vi "cam_entropy_trigger.vi"() -> ()   [LabVIEW 2015]
uses:
  <vilib>/userdefined/High Color/IMAQdx.ctl
  <vilib>/vision/driver/IMAQdx.llb/IMAQdx Acquisition Mode.ctl
  <vilib>/vision/driver/NI_Vision_Acquisition_Software.lvlib
  <vilib>/Analysis/NI_AALBase.lvlib
panel:
  in  "Image Name":string
  in  "File Path":path
  out "buffer #":u32
  out "loop count":i32
  in  "Manual Trigger":bool
  in  "error in":errorcluster
  in  "IMAQdx Session":T1="cam0"
  out "Camera Image":T2(plugin-control)
  in  "stop":bool
  out "Skip Frame":bool
  out "Trigger":bool
  out "Abs Entropy":dbl(graph)
  in  "Entropy Threshold":dbl=0.1
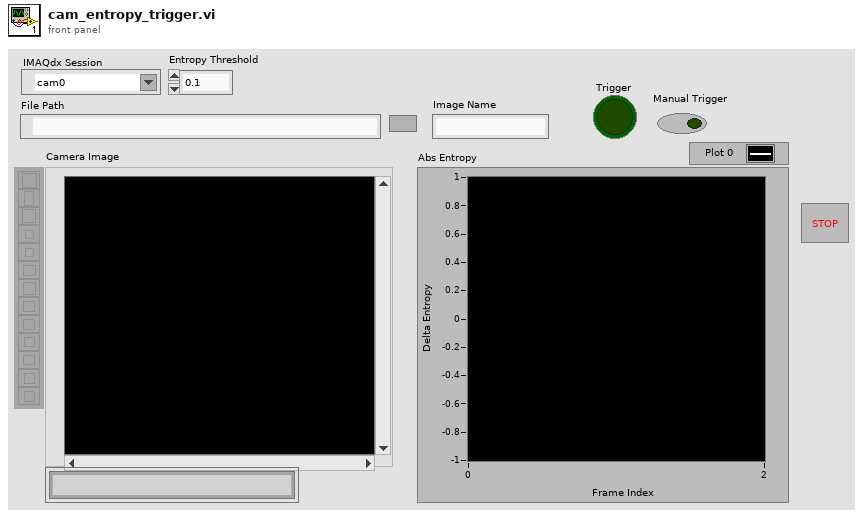
[diagram p1: front panel]
types:
  T1 = typedef "IMAQdx.ctl" = refnum<k21>
  T2 = typedef "IMAQ Image.ctl" = refnum<image>
  T3 = typedef "NI_Vision_Acquisition_Software.lvlib/IMAQdx Acquisition Mode.ctl" = enum32{"One Shot", "Continuous"}
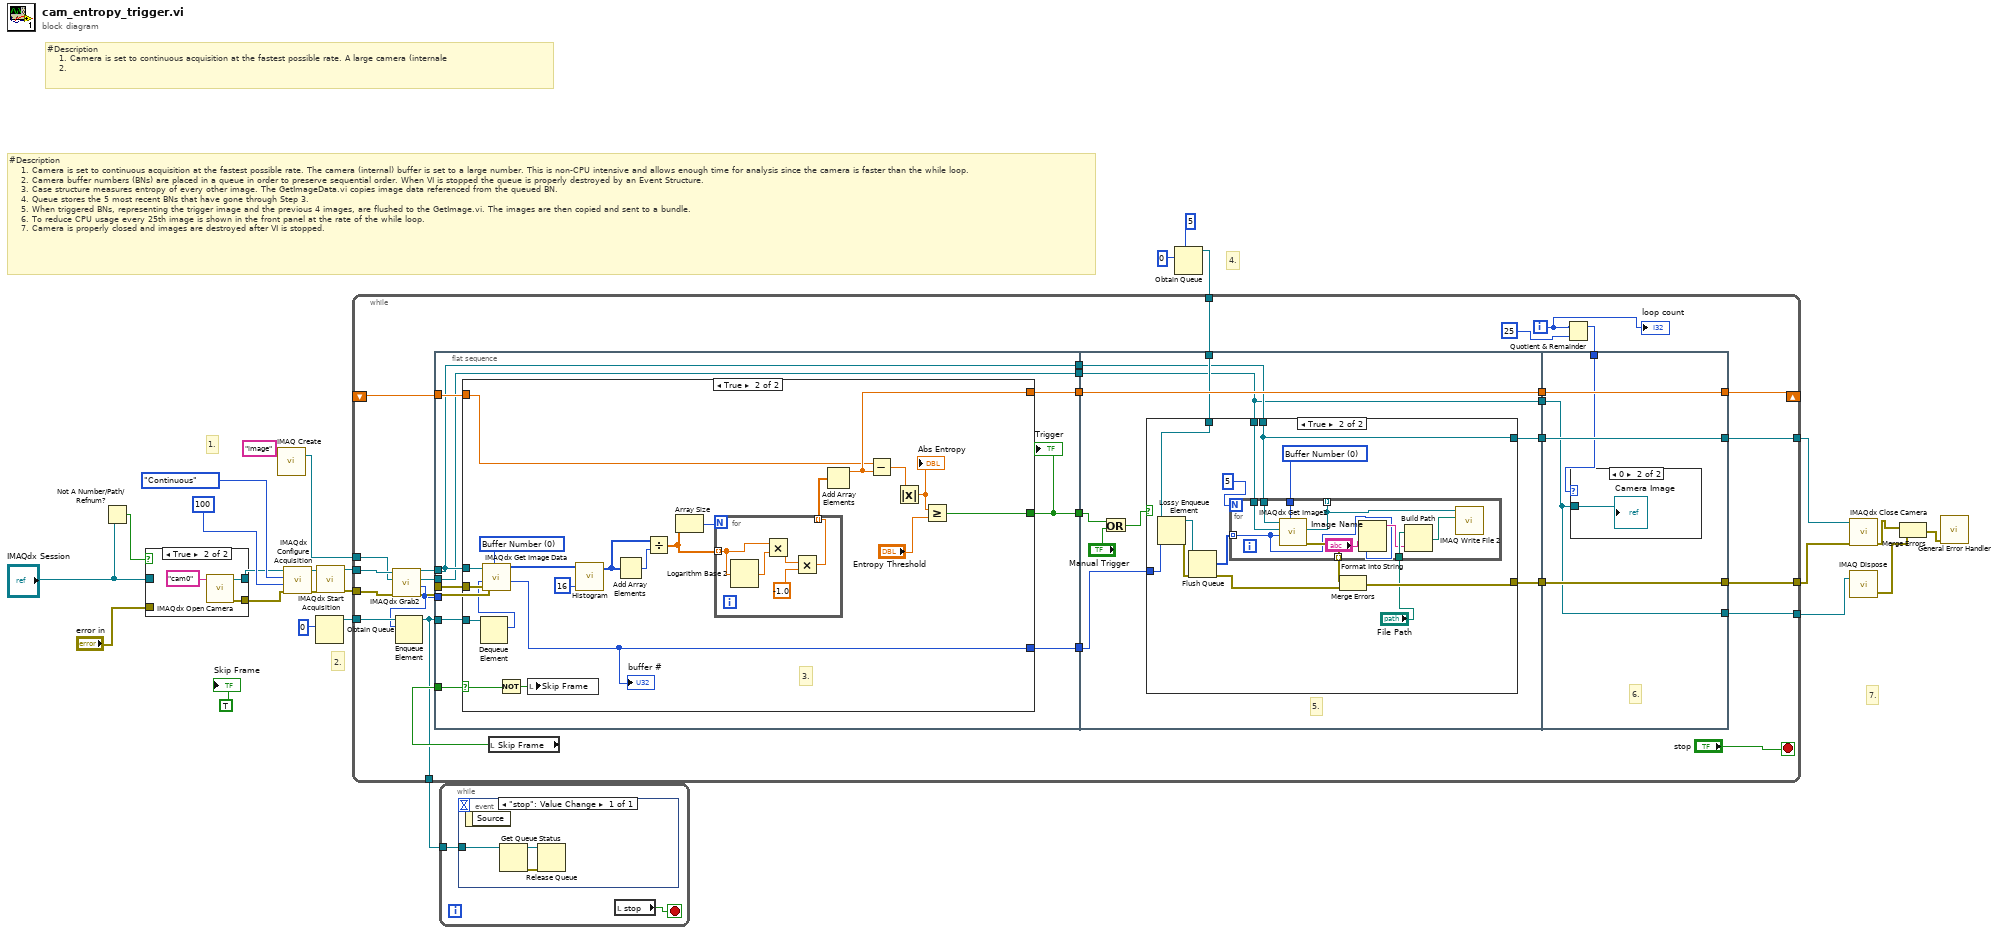
[diagram p0: block diagram]
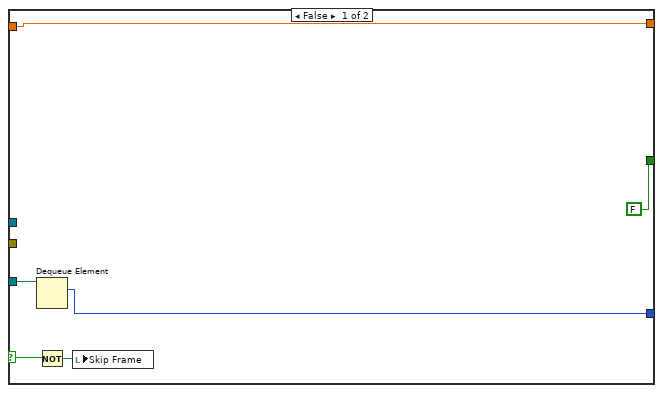
[diagram p3: hidden frame]
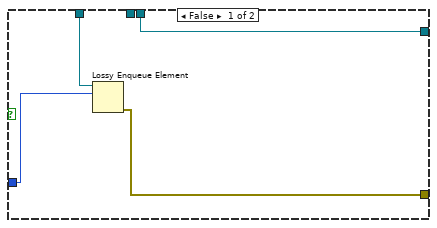
[diagram p4: hidden frame]
diagram:
  # "#Description\n    1. Camera is set to continuous acquisition at the fastest possible rate. The camera (internal) buffer is set to a large number. This is non-CPU intensive and allows enough time for analysis since the camera is faster than the while loop.\n    2. Camera buffer numbers (BNs) are placed in a queue in order to preserve sequential order. When VI is stopped the queue is properly destroyed by an Event Structure.\n    3. Case structure measures entropy of every other image. The GetImageData.vi copies image data referenced from the queued BN. \n    4. Queue stores the 5 most recent BNs that have gone through Step 3.\n    5. When triggered BNs, representing the trigger image and the previous 4 images, are flushed to the GetImage.vi. The images are then copied and sent to a bundle.\n    6. To reduce CPU usage every 25th image is shown in the front panel at the rate of the while loop.\n    7. Camera is properly closed and images are destroyed after VI is stopped."
  # "7."
  # "4."
  # "2."
  # "1."
  # "#Description\n    1. Camera is set to continuous acquisition at the fastest possible rate. A large camera (internale\n    2."
  n1 = Not A Number/Path/Refnum?(number/path/refnum="IMAQdx Session") -> (NaN/Path/Refnum?=w16:bool)
  n2 = case shown="True" w16 {
    tunnel: [w28 w31] -> w13
    tunnel: "IMAQdx Session" -> [w28 _]
    tunnel: [w27 w30] -> w12
    tunnel: "error in" -> [w27 _]
    frame False {
    }
    frame True {
      n3 = call <vilib>:"IMAQdx Open Camera.vi"("Session In"="cam0") -> ("error out"=w30:errorcluster, "Session Out"=w31:T1)  [unwired: 9 in]
    }
  }
  n4 = call "IMAQ Create"("Image Name"="image") -> ("New Image"=w7:T2)  [unwired: 4 in, 1 out]
  n5 = call <vilib>:"IMAQdx Configure Acquisition.vi"("error in"=w12, "Number of Buffers"=u32 100, "Continuous?"=IMAQdx_Acquisition_Mode."Continuous", "Session In"=w13) -> ("error out"=w18:errorcluster, "Session Out"=w19:T1)  [unwired: 6 in]
  n6 = Obtain Queue(element data type=0) -> (queue out=w22:refnum<queue>)  [unwired: 4 in, 2 out]
  n7 = call <vilib>:"IMAQdx Start Acquisition.vi"("error in"=w18, "Session In"=w19) -> ("error out"=w9:errorcluster, "Session Out"=w11:T1)  [unwired: 8 in]
  n8 = Obtain Queue(max queue size (-1, unlimited)=5, element data type=0) -> (queue out=w24:refnum<queue>)  [unwired: 3 in, 2 out]
  n9 = while {
    tunnel: w11 -> [w59]
    tunnel: w9 -> [w58]
    shift-right: [w57] -> _
    shift-left: _ -> [w56]
    tunnel: w24 -> [w53]
    tunnel: w22 -> [w51]
    tunnel: [w44] -> w21
    tunnel: [w43] -> w20
    tunnel: w7 -> [w36]
    tunnel: [w34] -> w5
    tunnel: [w33] -> w4
    i -> [w32]
    stop <- "stop" stop-if-true
    n10 = call <vilib>:"IMAQdx Grab2.vi"("error in"=w58, "Image In"=w36, "Session In"=w59) -> ("error out"=w60:errorcluster, "Buffer Number Out"=w35:u32, "Image Out"=w46:T2, "Session Out"=w47:T1)  [unwired: 5 in]
    n11 = Enqueue Element(queue=w51, element=w35) -> (queue out=w43:refnum<queue>)  [unwired: 2 in, 2 out]
    n12 = flat-sequence {
      tunnel: w60 -> [w69]
      tunnel: w56 -> [w67]
      tunnel: w55 -> [w66]
      tunnel: [w68] -> w54
      tunnel: w47 -> [w62]
      tunnel: [w65] -> w52
      tunnel: w43 -> [w64]
      tunnel: [w63] -> w49
      tunnel: [w62] -> w48
      tunnel: w46 -> [w61]
      tunnel: [w61] -> w45
      tunnel: w35 -> [_]
      tunnel: w54 -> [w111]
      tunnel: w53 -> [w110]
      tunnel: w52 -> [w109]
      tunnel: w49 -> [w104]
      tunnel: w48 -> [w108]
      tunnel: w45 -> [w105]
      tunnel: [w111] -> w42
      tunnel: [w107] -> w41
      tunnel: [w106] -> w40
      tunnel: [w105] -> w37
      tunnel: [w141] -> w44
      tunnel: [w142] -> w34
      tunnel: [w143] -> w57
      tunnel: w42 -> [w143]
      tunnel: w41 -> [w142]
      tunnel: w40 -> [w141]
      tunnel: w38 -> [w140]
      tunnel: w37 -> [w139]
      tunnel: [w139] -> w33
      frame #0 {
        n13 = case shown="True" w66 {
          selector: w66 -> [w74 w85]
          tunnel: w69 -> [_ w81]
          tunnel: [w75 w87] -> w68
          tunnel: w67 -> [w75 w86]
          tunnel: [FALSE w83] -> w63
          tunnel: w62 -> [_ w82]
          tunnel: [w70 w77] -> w65
          tunnel: w64 -> [w71 w79]
          frame False {
            n14 = Dequeue Element(queue=w71) -> (element=w70:i32)  [unwired: 2 in, 3 out]
            n15 = Not(x=w74) -> (.not. x?=w73:bool)
            n16 = local write "Skip Frame"(w73) -> ()
          }
          frame True {
            w78 = u16 0 items=["Buffer Number"]
            # "3."
            n17 = Dequeue Element(queue=w79) -> (element=w76:i32)  [unwired: 2 in, 3 out]
            n18 = call <vilib>:"IMAQdx Get Image Data.vi"("Buffer Number Mode (Next)"=w78, "error in"=w81, "Buffer Number In"=w76, "Session In"=w82) -> ("Buffer Number Out"=w77:u32, "Image Data Array"=w80:u8[])  [unwired: 4 in, 2 out]
            "buffer #" <- w77
            n19 = Not(x=w85) -> (.not. x?=w84:bool)
            n20 = local write "Skip Frame"(w84) -> ()
            n21 = call <vilib>:"Histogram.vi"("intervals"=16, "X"=w80) -> ("Histogram: h(x)"=w92:i32[])  [unwired: 6 in, 3 out]
            n22 = Add Array Elements(numeric array=w92) -> (sum=w93:i32)
            n23 = Divide(x=w92, y=w93) -> (x/y=w96:dbl[])
            n24 = Array Size(array=w96) -> (size(s)=w95:i32)
            n25 = for {
              N: w95 -> [_]
              tunnel: w96 -> [w98] mode=indexing
              tunnel: [w97] -> w90 mode=indexing
              n26 = Logarithm Base 2(1:w98) -> (0:w99:dbl)
              n27 = Multiply(x=w98, y=w99) -> (x*y=w100:dbl)
              n28 = Multiply(x=w100, y=-1.0) -> (x*y=w97:dbl)
            }
            n29 = Add Array Elements(numeric array=w90) -> (sum=w87:dbl)
            n30 = Subtract(x=w86, y=w87) -> (x-y=w91:dbl)
            n31 = Absolute Value(x=w91) -> (abs(x)=w88:dbl)
            "Abs Entropy" <- w88
            n32 = Greater Or Equal?(x=w88, y="Entropy Threshold") -> (x >= y?=w83:bool)
          }
        }
        "Trigger" <- w63
      }
      frame #1 {
        # "5."
        n33 = Or(x=w104, y="Manual Trigger") -> (x .or. y?=w103:bool)
        n34 = case shown="True" w103 {
          tunnel: [w113 w127] -> w107
          tunnel: w110 -> [w115 w122]
          tunnel: w109 -> [w114 w123]
          tunnel: w108 -> [w112 w118]
          tunnel: w105 -> [_ w119]
          tunnel: [w112 w118] -> w106
          frame False {
            n35 = Lossy Enqueue Element(queue=w115, element=w114) -> (error out=w113:errorcluster)  [unwired: 1 in, 3 out]
          }
          frame True {
            w124 = u16 0 items=["Buffer Number"]
            n36 = Lossy Enqueue Element(queue=w122, element=w123) -> (queue out=w121:refnum<queue>, error out=w120:errorcluster)  [unwired: 1 in, 2 out]
            n37 = Flush Queue(queue=w121, error in (no error)=w120) -> (remaining elements=w126:i32[], error out=w128:errorcluster)  [unwired: 1 out]
            n38 = for {
              N: 5 -> [_]
              tunnel: [w134] -> _ mode=indexing
              tunnel: w126 -> [w129] mode=indexing
              tunnel: [w138] -> w125 mode=indexing
              tunnel: w124 -> [w137]
              tunnel: w118 -> [w136]
              tunnel: w119 -> [w135]
              tunnel: "File Path" -> [w131]
              n39 = call <vilib>:"IMAQdx Get Image2.vi"("Buffer Number Mode (Next)"=w137, "Buffer Number In"=w129, "Image In"=w135, "Session In"=w136) -> ("error out"=w138:errorcluster, "Image Out"=w134:T2)  [unwired: 4 in, 2 out]
              n40 = Format Into String("Image Name", w129) -> (resulting string=w130:string)  [unwired: 3 in, 1 out]
              n41 = Build Path(base path=w131, name or relative path=w130) -> (appended path=w132:path)
              n42 = call-poly "IMAQ Write File 2"("File Path"=w132, "Image"=w134) -> ()  [unwired: 8 in, 2 out]
            }
            n43 = Merge Errors(w125, w128) -> (w127:errorcluster)
          }
        }
      }
      frame #2 {
        # "6."
        n44 = case shown="0" w140 {
          tunnel: w139 -> [_ w144]
          frame 1.., Default {
            # "#Only previewing\non every multiple"
          }
          frame 0 {
            "Camera Image" <- w144
          }
        }
      }
    }
    n45 = local read "Skip Frame"() -> (w55:bool)
    n46 = Quotient & Remainder(x=w32, y=25) -> (x-y*floor(x/y)=w38:i32)  [unwired: 1 out]
    "loop count" <- w32
  }
  n47 = while {
    tunnel: w20 -> [w146]
    stop <- w145 stop-if-true
    n48 = event shown="[0] \"stop\": Value Change" {
      selector: _ -> [_]
      dyn-events: _ -> [_]
      timeout: _ -> [_]
      tunnel: w146 -> [w147]
      event "stop": Value Change {
        n49 = event-data() -> ()  [unwired: 1 in, 1 out]
        n50 = Get Queue Status(queue=w147) -> (queue out=w148:refnum<queue>, error out=w149:errorcluster)  [unwired: 2 in, 6 out]
        n51 = Release Queue(queue=w148, error in (no error)=w149) -> ()  [unwired: 1 in, 3 out]
      }
    }
    n52 = local read "stop"() -> (w145:bool)
  }
  n53 = call <vilib>:"IMAQdx Close Camera.vi"("error in"=w5, "Session In"=w21) -> ("error out"=w1:errorcluster)  [unwired: 9 in]
  n54 = call "IMAQ Dispose"("Image"=w4) -> ("error out"=w2:errorcluster)  [unwired: 5 in]
  n55 = Merge Errors(w1, w2) -> (w3:errorcluster)
  n56 = call <vilib>:"General Error Handler.vi"("error in (no error)"=w3) -> ()  [unwired: 4 in, 11 out]
  "Skip Frame" <- TRUE
